vi "Main_Initialize.vi"(8 "error in":errorcluster, 11 "VI Refnum":refnum<vi>) -> (0 "error out":errorcluster, 3 "Main Data Buffer":T1)   [LabVIEW 2020, in "SECS Bridge.lvlib"]
uses:
  SECS Bridge.lvlib
  Main Data Buffer.ctl
  SECS Communication/HSMS Class/HSMS Class.lvclass
  SECS Communication/SECS Data Class/SECS Data Class.lvclass
  SECS Scenarios/Scenarios Class/Scenarios Class.lvclass
  SECS Communication/SECS-II Class/SECS-II Class.lvclass
  SECS Communication/HSMS Class/Notifier Data.ctl
  SECS Communication/HSMS Class/Notifier Type.ctl
  SECS Scenarios/Scenarios Class/Broadcast Refnum.ctl
  SECS Scenarios/Scenarios Class/13-EnableDisable Alarm.ctl
  SECS Scenarios/Scenarios Class/15-Process Program Request.ctl
  SECS Scenarios/Scenarios Class/16-Process Program Send.ctl
  SECS Communication/S7 Message Class/S7F4.ctl
  SECS Scenarios/Scenarios Class/17-Deleting a Process Program by Host.ctl
  SECS Communication/S7 Message Class/S7F18.ctl
  SECS Scenarios/Scenarios Class/18-Host Requests Equipment Process Program Directory.ctl
  SECS Scenarios/Scenarios Class/19-Equipment Process Program Uploading.ctl
  SECS Communication/SECS-II Class/Format Code.ctl
  SECS Scenarios/Scenarios Class/20[1]-Process Program Downloading.ctl
  SECS Communication/S7 Message Class/S7F2.ctl
  SECS Scenarios/Scenarios Class/20[2]-Process Program Downloading.ctl
  SECS Communication/S7 Message Class/S7F23.ctl
  SECS Communication/S7 Message Class/S7F24.ctl
  SECS Scenarios/Scenarios Class/22-Host Sends Information to Equipment.ctl
  SECS Communication/S10 Message Class/S10F4.ctl
  SECS Scenarios/Scenarios Class/26-Host Requests to Enter OFF-Line.ctl
  SECS Scenarios/Scenarios Class/27-Host Requests to Enter On-Line.ctl
  SECS Communication/S1 Message Class/S1F18.ctl
  SECS Scenarios/Scenarios Class/28[1]-Remote Control[PP-SELECT].ctl
  SECS Scenarios/Scenarios Class/28[2]-Remote Control[START].ctl
  SECS Scenarios/Scenarios Class/28[3]-Remote Control[STOP].ctl
  SECS Scenarios/Scenarios Class/28[4]-Remote Control[LOCAL].ctl
  SECS Scenarios/Scenarios Class/28[5]-Remote Control[REMOTE].ctl
  SECS Scenarios/Scenarios Class/28[6]-Remote Control[RCMD].ctl
  SECS Communication/S2 Message Class/S2F41.ctl
  SECS Communication/S2 Message Class/S2F42.ctl
  SECS Scenarios/Scenarios Class/30-Host Requests Equipment to Set Time.ctl
  SECS Communication/S2 Message Class/S2F32.ctl
  SECS Scenarios/Scenarios Class/31-Host Requests Time Value from Equipment.ctl
  SECS Scenarios/Scenarios Class/32[1]-Trace Data Collection.ctl
  SECS Scenarios/Scenarios Class/32[2]-Trace Data Collection.ctl
  SECS Communication/S2 Message Class/S2F24.ctl
  File FGV Method.ctl
  SECS Communication/HSMS Class/Role.ctl
  SECS Communication/HSMS Class/HSMS Class.lvclass/HSMS Class.ctl
  SECS Communication/HSMS Class/Write Log Path.vi
  SECS Communication/HSMS Class/Write Session ID.vi
  SECS Communication/HSMS Class/Write T3(Reply Timeout).vi
  SECS Communication/HSMS Class/Write T5(Separation Timeout).vi
  SECS Communication/HSMS Class/Write T6(Control Timeout).vi
  SECS Communication/HSMS Class/Write T7(Not Selected Timeout).vi
  SECS Communication/HSMS Class/Write T8(Inter-Character Timeout).vi
  SECS Communication/HSMS Class/Read Recive User Event.vi
  SECS Communication/HSMS Class/Read Notifier User Event.vi
  PPL/Universal Function.lvlibp
  SECS Communication/S2 Message Class/S2 Message Class.lvclass
  SECS Communication/S1 Message Class/S1 Message Class.lvclass
  SECS Communication/S10 Message Class/S10 Message Class.lvclass
  SECS Communication/S7 Message Class/S7 Message Class.lvclass
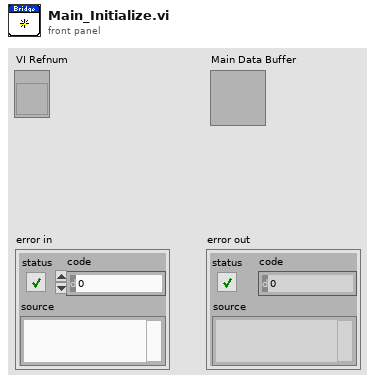
[diagram p1: front panel]
types:
  T1 = typedef "SECS Bridge.lvlib/Main Data Buffer.ctl" = cluster{"HSMS Class":refnum<class "HSMS Class.lvclass">, "SECS Data Class":refnum<class "SECS Data Class.lvclass">, "Scenarios Class":refnum<class "Scenarios Class.lvclass">, "VI Refnum":refnum<vi>, "Ctl Refnum Map":map{string, refnum<vi>}, "Timeout":i32, "Notifier Data":string[], "Event Refnum":refnum<event-registration>}
  T2 = typedef "SECS Scenarios.lvlib/Scenarios Class.lvclass/Broadcast Refnum.ctl" = cluster{"13-EnableDisable Alarm":refnum<user-event>, "15-Process Program Request":refnum<user-event>, "16-Process Program Send":refnum<user-event>, "17-Deleting a Process Program by Host":refnum<user-event>, "18-Host Requests Equipment Process Program Directory":refnum<user-event>, "19-Equipment Process Program Uploading":refnum<user-event>, "20[1]-Process Program Downloading":refnum<user-event>, "20[2]-Process Program Downloading":refnum<user-event>, "22-Host Sends Information to Equipment":refnum<user-event>, "26-Host Requests to Enter OFF-Line":refnum<user-event>, "27-Host Requests to Enter On-Line":refnum<user-event>, "28[1]-Remote Control[PP-SELECT]":refnum<user-event>, "28[2]-Remote Control[START]":refnum<user-event>, "28[3]-Remote Control[STOP]":refnum<user-event>, "28[4]-Remote Control[LOCAL]":refnum<user-event>, "28[5]-Remote Control[REMOTE]":refnum<user-event>, "28[6]-Remote Control[RCMD]":refnum<user-event>, "30-Host Requests Equipment to Set Time":refnum<user-event>, "31-Host Requests Time Value from Equipment":refnum<user-event>, "32[1]-Trace Data Collection":refnum<user-event>, "32[2]-Trace Data Collection":refnum<user-event>}
  T3 = typedef "SECS Communication.lvlib/HSMS Class.lvclass/Role.ctl" = enum16{"Passive", "Active"}
  T4 = typedef "SECS Bridge.lvlib/File FGV Method.ctl" = enum16{"Get", "Put", "Read", "Write"}
  T5 = typedef "SECS Bridge.lvlib/Configuration.ctl" = cluster{"T3(Reply Timeout)":i32, "T5(Separation Timeout)":i32, "T6(Control Timeout)":i32, "T7(Not Selected Timeout)":i32, "T8(Inter-Character Timeout)":i32, "Session ID":u16, "Log Path":path, "IP Address":string, "Port":u16}
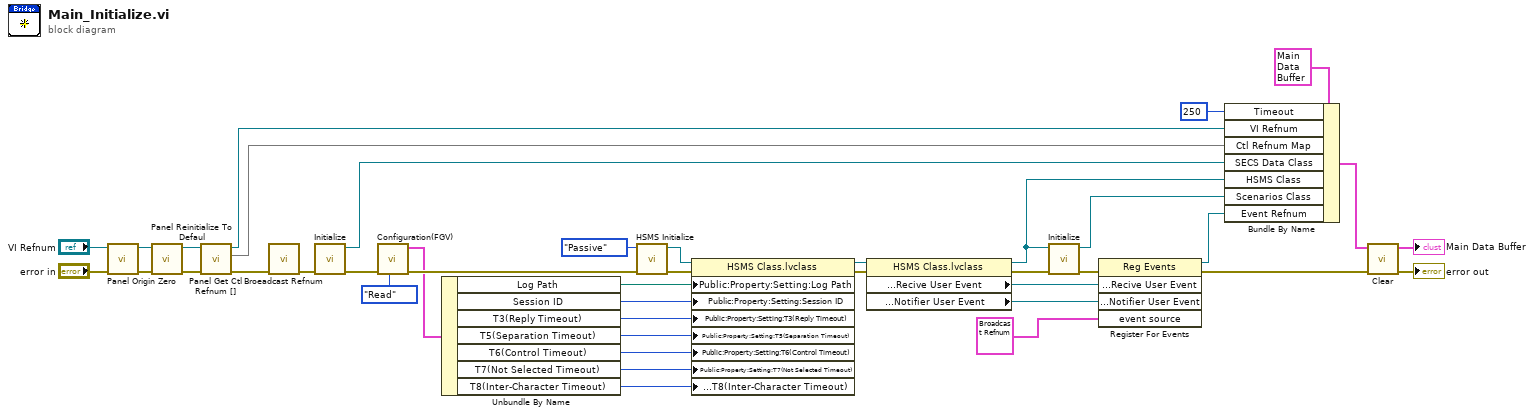
[diagram p0: block diagram]
diagram:
  n1 = call "Panel Origin Zero.vi"("error in"="error in", "VI Refnum In"="VI Refnum") -> ("error out"=w38:errorcluster, "VI Refnum Out"=w39:refnum<vi>)  [unwired: 8 in]
  n2 = call "Panel Reinitialize To Defaul.vi"("error in"=w38, "VI Refnum In"=w39) -> ("error out"=w36:errorcluster, "VI Refnum Out"=w37:refnum<vi>)  [unwired: 8 in]
  n3 = call "Panel Get Ctl Refnum [].vi"("error in"=w36, "VI Refnum In"=w37) -> ("error out"=w5:errorcluster, "Ctl Refnum Map"=w32:map{string, refnum<vi>}, "VI Refnum Out"=w33:refnum<vi>)  [unwired: 7 in]
  n4 = call "Broeadcast Refnum.vi"("error in"=w5) -> ("error out"=w4:errorcluster)  [unwired: 9 in, 1 out]
  n5 = call "Initialize.vi"("error in"=w4) -> ("error out"=w29:errorcluster, "SECS Data Class out"=w16:refnum<class "SECS Data Class.lvclass">)  [unwired: 9 in]
  n6 = call "Configuration(FGV).vi"("File FGV Method"=File_FGV_Method."Read", "error in"=w29) -> ("error out"=w28:errorcluster, "Configuration Out"=w26:T5)  [unwired: 8 in]
  n7 = Unbundle By Name(w26) -> ("Log Path"=w23:path, "Session ID"=w22:u16, "T3(Reply Timeout)"=w21:i32, "T5(Separation Timeout)"=w20:i32, "T6(Control Timeout)"=w19:i32, "T7(Not Selected Timeout)"=w18:i32, "T8(Inter-Character Timeout)"=w17:i32)
  n8 = call "HSMS Initialize.vi"("error in (no error)"=w28, "Role"=Role."Passive") -> ("error out"=w27:errorcluster, "HSMS Class out"=w31:refnum<class "HSMS Class.lvclass">)  [unwired: 8 in]
  n9 = property class="HSMS Class.lvclass"(reference=w31, error in=w27, "Public:Property:Setting:Log Path"=w23, "Public:Property:Setting:Session ID"=w22, "Public:Property:Setting:T3(Reply Timeout)"=w21, "Public:Property:Setting:T5(Separation Timeout)"=w20, "Public:Property:Setting:T6(Control Timeout)"=w19, "Public:Property:Setting:T7(Not Selected Timeout)"=w18, "Public:Property:Setting:T8(Inter-Character Timeout)"=w17) -> (reference out=w25:refnum<class "HSMS Class.lvclass">, error out=w24:errorcluster)
  n10 = property class="HSMS Class.lvclass"(reference=w25, error in=w24) -> (reference out=w11:refnum<class "HSMS Class.lvclass">, error out=w15:errorcluster, "Public:Property:User Event:Recive User Event"=w12:refnum<user-event>, "Public:Property:User Event:Notifier User Event"=w10:refnum<user-event>)
  n11 = call "Initialize.vi"("error in (no error)"=w15, "HSMS Class"=w11) -> ("error out"=w13:errorcluster, "Scenarios Class out"=w14:refnum<class "Scenarios Class.lvclass">)  [unwired: 8 in]
  n12 = register-events(error in=w13, w12, w10, T2 {"13-EnableDisable Alarm"=refnum, "15-Process Program Request"=refnum, "16-Process Program Send"=refnum, "17-Deleting a Process Program by Host"=refnum, "18-Host Requests Equipment Process Program Directory"=refnum, "19-Equipment Process Program Uploading"=refnum, "20[1]-Process Program Downloading"=refnum, "20[2]-Process Program Downloading"=refnum, "22-Host Sends Information to Equipment"=refnum, "26-Host Requests to Enter OFF-Line"=refnum, "27-Host Requests to Enter On-Line"=refnum, "28[1]-Remote Control[PP-SELECT]"=refnum, "28[2]-Remote Control[START]"=refnum, "28[3]-Remote Control[STOP]"=refnum, "28[4]-Remote Control[LOCAL]"=refnum, "28[5]-Remote Control[REMOTE]"=refnum, "28[6]-Remote Control[RCMD]"=refnum, "30-Host Requests Equipment to Set Time"=refnum, "31-Host Requests Time Value from Equipment"=refnum, "32[1]-Trace Data Collection"=refnum, "32[2]-Trace Data Collection"=refnum} ("event source")) -> (reference out=w2:refnum<event-registration>, error out=w9:errorcluster)  [unwired: 1 in]
  n13 = Bundle By Name(cluster=T1 {"HSMS Class"=refnum, "SECS Data Class"=refnum, "Scenarios Class"=refnum, "VI Refnum"=refnum, "Ctl Refnum Map"={}, "Timeout"=0, "Notifier Data"=[], "Event Refnum"=refnum} ("Main Data Buffer"), "Timeout"=250, "VI Refnum"=w33, "Ctl Refnum Map"=w32, "SECS Data Class"=w16, "HSMS Class"=w11, "Scenarios Class"=w14, "Event Refnum"=w2) -> (w8:T1)
  n14 = call "Clear.vi"("error in"=w9, "Main Data Buffer In"=w8) -> ("error out"=→"error out":errorcluster, "Main Data Buffer Out"=→"Main Data Buffer":T1)  [unwired: 8 in]
